vi "FlagInstance-Update GEvt Refs.vi"(10 "Error in":errorcluster caption="Error in (no error)") -> (2 "Error out":errorcluster, 3 "New Random Change Flag":u64=4603270806574966694 format="%08x")   [LabVIEW 2017, in "Communicable State Machine.lvlib"]
uses:
  Communicable State Machine.lvlib
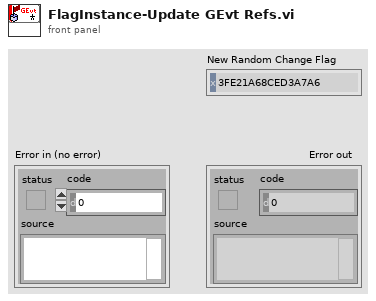
[diagram p1: front panel]
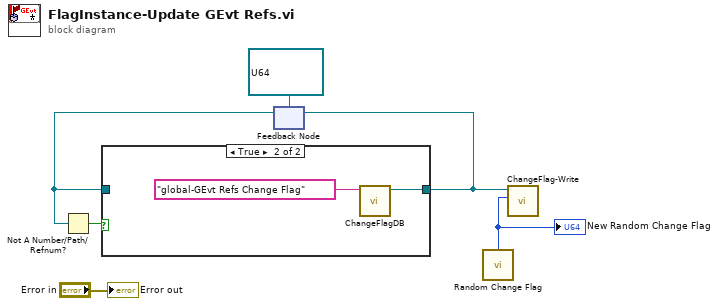
[diagram p0: block diagram]
diagram:
  n1 = feedback #1(refnum<queue> refnum ("ChangeFlagQ")) -> (w4:refnum<queue>)
  n2 = Not A Number/Path/Refnum?(number/path/refnum=w4) -> (NaN/Path/Refnum?=w5:bool)
  n3 = case shown="True" w5 {
    tunnel: [w7 w8] -> w2
    tunnel: w4 -> [w7 _]
    frame False {
    }
    frame True {
      n4 = call "ChangeFlagDB.vi"("ChangeFlagName"="global-GEvt Refs Change Flag" ("global-CSMQ FGV Change Flag")) -> ("ChangeFlagQ"=w8:refnum<queue>)  [unwired: 10 in]
    }
  }
  n5 = feedback-in #1(w2) -> ()
  n6 = call "Random Change Flag.vi"() -> ("Random Change Flag"=w1:u64)  [unwired: 2 in]
  "New Random Change Flag" <- w1
  n7 = call "ChangeFlag-Write.vi"("ChangeFlag"=w1, "ChangeFlagQ"=w2) -> ()  [unwired: 9 in, 1 out]
  "Error out" <- "Error in"
